vi "NI 9203 DOUBLE TASK.vi"(0 "MODULE 1 (4-20mA)":string, 1 "MODULE 2 (4-20mA)":string, 2 "sample mode":i32(ring)=10178 items=["Finite Samples"=10178, "Continuous Samples"=10123, "Hardware Timed Single Point"=12522], 4 "rate":dbl=1000.0 format="%0.2f", 5 "error in":errorcluster) -> (14 "task out":refnum<k21>, 19 "error out":errorcluster)   [LabVIEW 2019]
uses:
  <vilib>/DAQmx/configure/timing.llb/DAQmx Timing (Sample Clock).vi
panel:
  out "error out 2":errorcluster
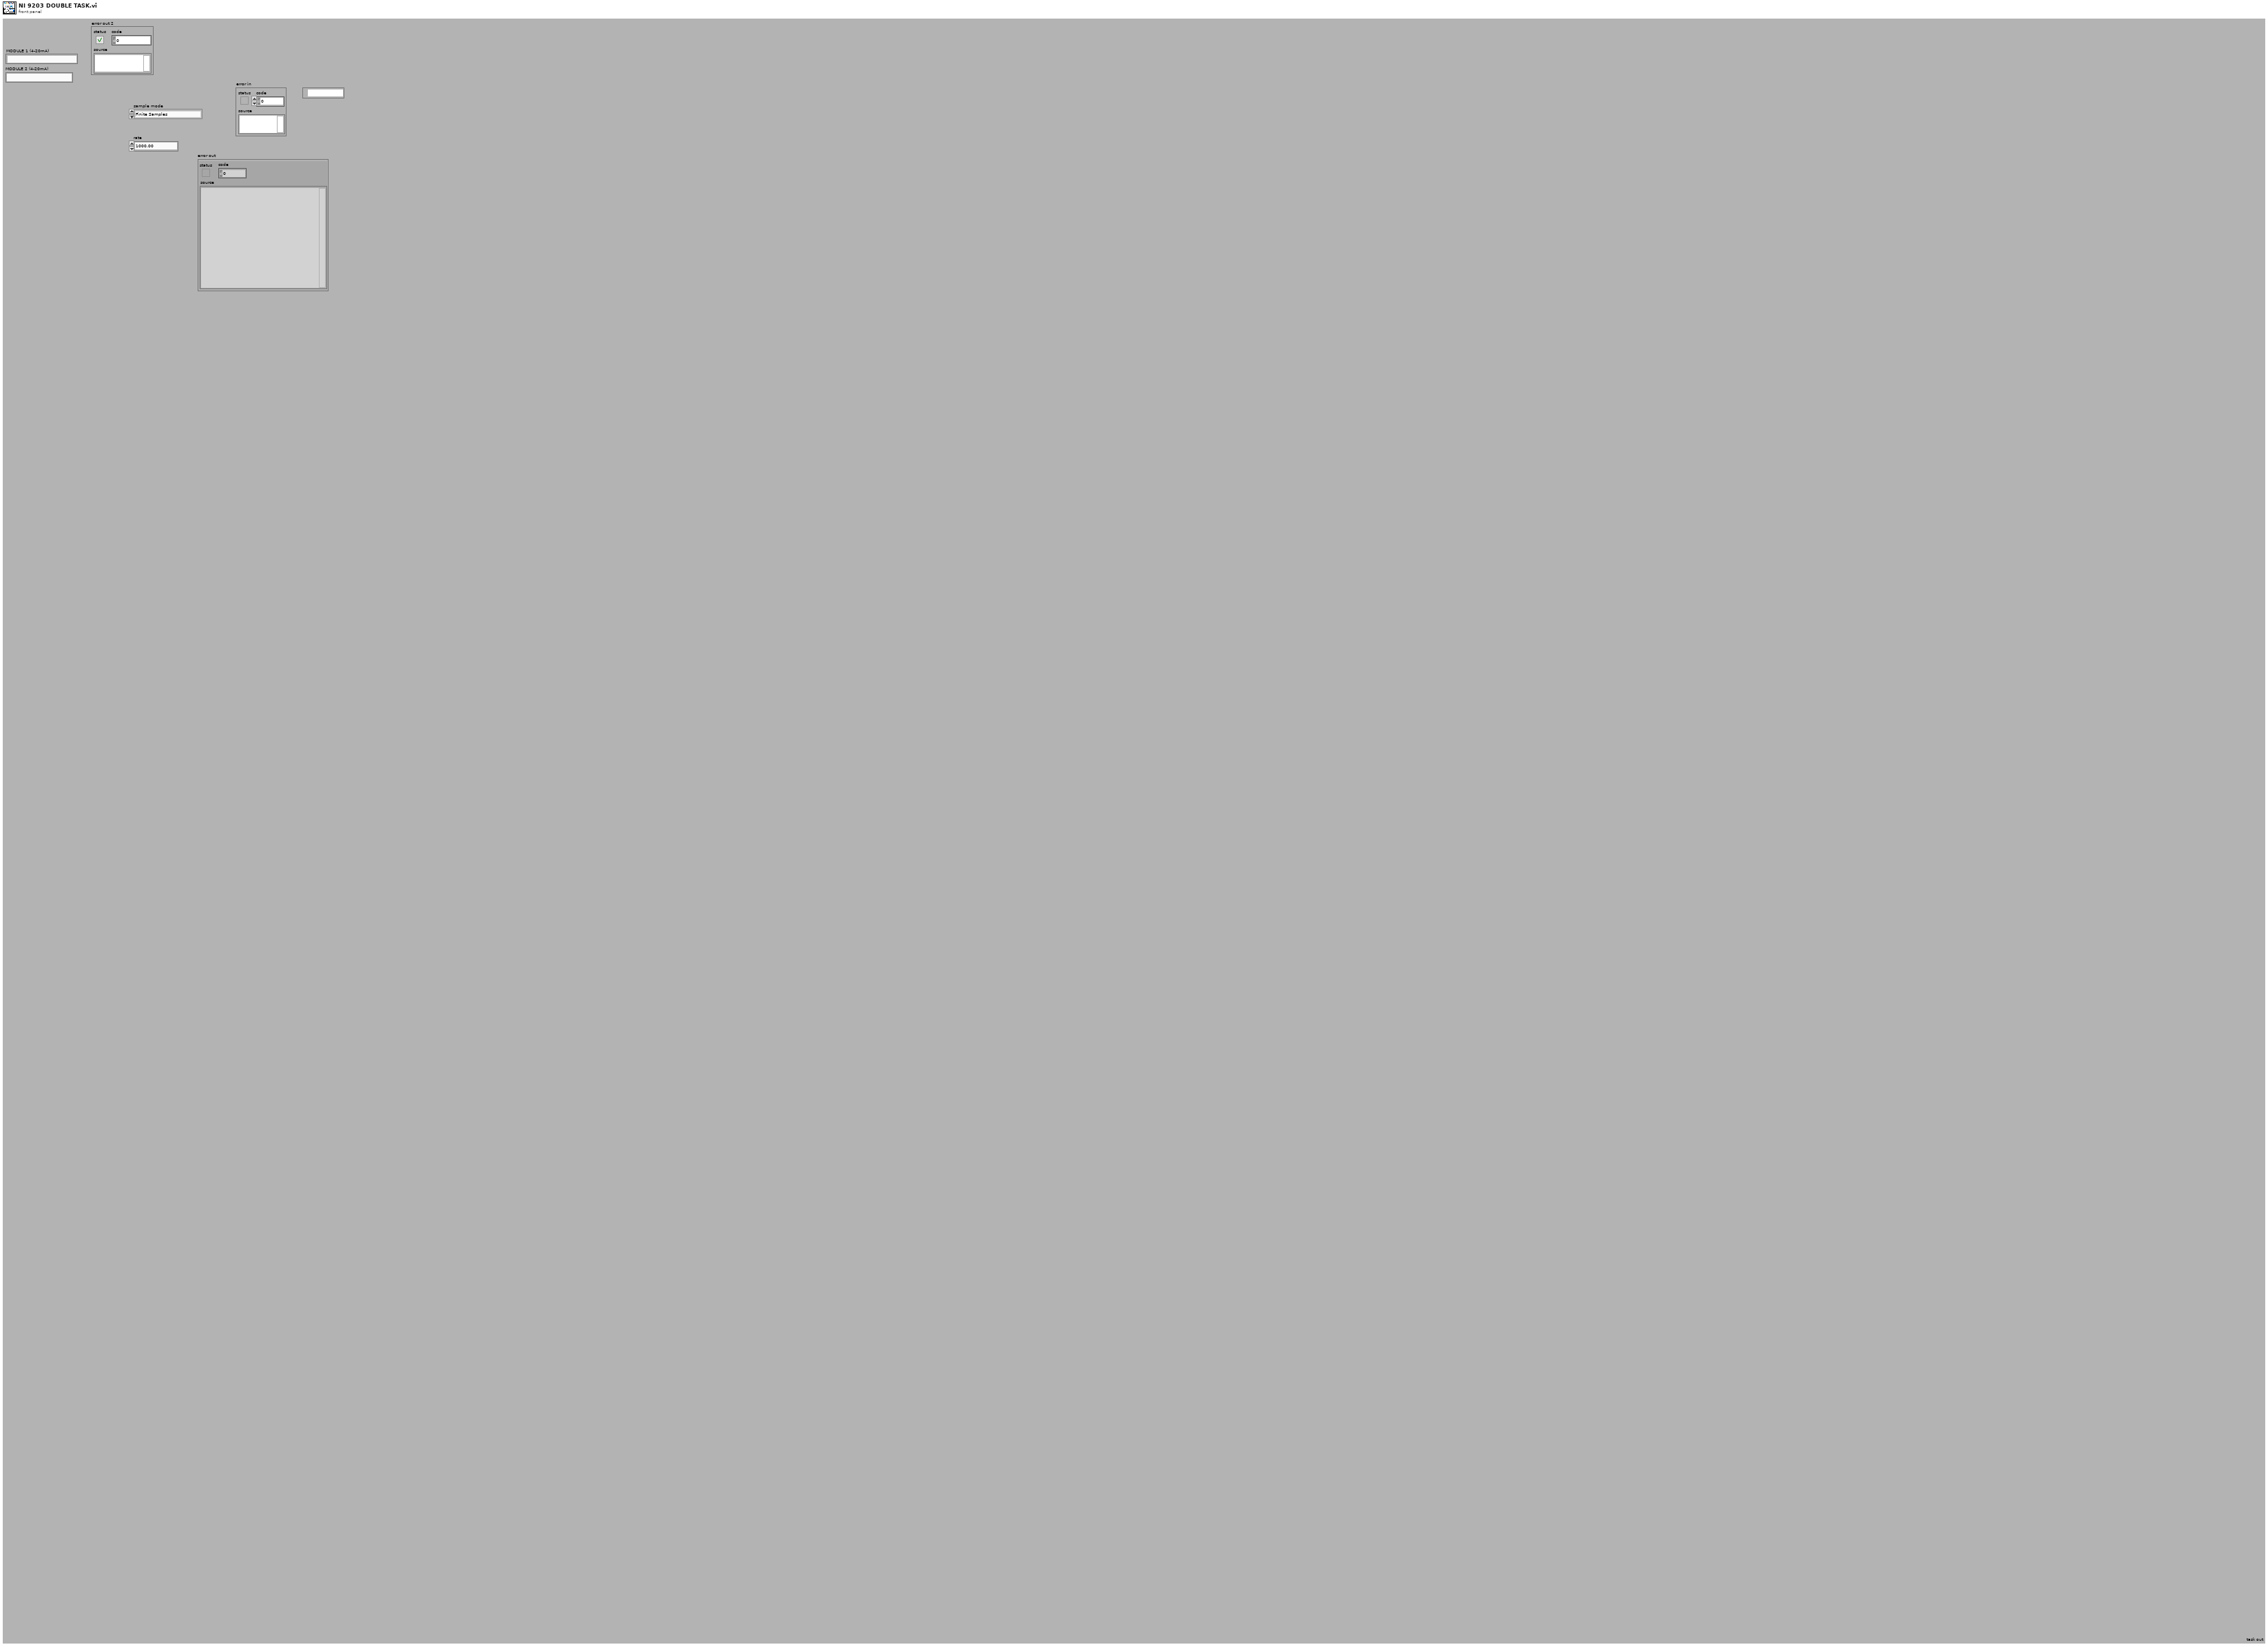
[diagram p1: front panel]
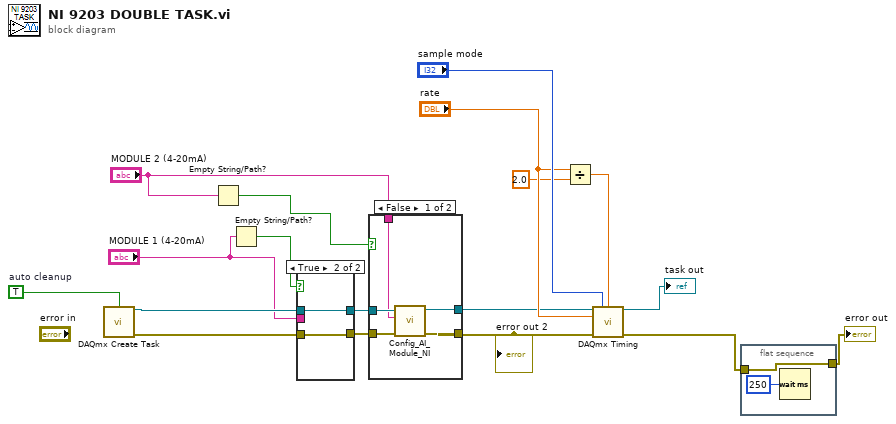
[diagram p0: block diagram]
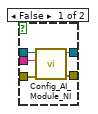
[diagram p2: hidden frame]
diagram:
  w17 = TRUE  # auto cleanup
  n1 = call <vilib>:"DAQmx Create Task.vi"("auto cleanup"=w17) -> ("task out"=w5:refnum<k21>, "error out"=w18:errorcluster)  [unwired: 13 in]
  n2 = Empty String/Path?(string/path="MODULE 2 (4-20mA)") -> (empty?=w3:bool)
  n3 = Empty String/Path?(string/path="MODULE 1 (4-20mA)") -> (empty?=w1:bool)
  n4 = case shown="True" w1 {
    tunnel: w18 -> [w23 w24]
    tunnel: w5 -> [w22 w25]
    tunnel: "MODULE 1 (4-20mA)" -> [w21 _]
    tunnel: [w20 w25] -> w9
    tunnel: [w19 w24] -> w8
    frame False {
      n5 = call "Config_AI_Module_NI.vi"("error in (no error)"=w23, "MODULE NAME"=w21, "Refnum in"=w22) -> ("error out"=w19:errorcluster, "Refnum out"=w20:refnum<k21>)  [unwired: 7 in]
    }
    frame True {
    }
  }
  n6 = case shown="False" w3 {
    tunnel: w9 -> [w30 w32]
    tunnel: w8 -> [w29 w31]
    tunnel: [w28 w32] -> w4
    tunnel: [w27 w31] -> w7
    tunnel: "MODULE 2 (4-20mA)" -> [w26 _]
    frame False {
      n7 = call "Config_AI_Module_NI.vi"("error in (no error)"=w29, "MODULE NAME"=w26, "Refnum in"=w30) -> ("error out"=w27:errorcluster, "Refnum out"=w28:refnum<k21>)  [unwired: 7 in]
    }
    frame True {
    }
  }
  "error out 2" <- w7
  n8 = Divide(x="rate", y=2.0) -> (x/y=w12:dbl)
  n9 = call-poly <vilib>:"DAQmx Timing.vi"("task/channels in"=w4, "sample mode"="sample mode", "samples per channel"=w12, "rate"="rate", "error in"=w7) -> ("task out"=→"task out":refnum<k21>, "error out"=w11:errorcluster)  [unwired: 9 in]
  n10 = flat-sequence {
    tunnel: [w33] -> w10
    tunnel: w11 -> [w33]
    frame #0 {
      n11 = Wait (ms)(milliseconds to wait=u32 250) -> ()  [unwired: 1 out]
    }
  }
  "error out" <- w10
